vi "letak-cube.vi"   [LabVIEW 2016, in "Moving Motor.lvrbt"]
uses:
  Moving Motor.lvrbt
  <vilib>/NXT/Hardware/Plugins/Tetrix 180 deg Servo/Tetrix180ServoAddress.ctl
  <vilib>/NXT/Hardware/Plugins/Tetrix DC Motor/TetrixDCMotorAddress.ctl
  <vilib>/NXT/NXTIO Xnodes/NXTIONodeSubVIs/TETRIX IO Move Servos.vi
  <vilib>/NXT/NXTIO Xnodes/NXTIONodeSubVIs/TETRIX IO Move DC Motors.vi
  <vilib>/NXT/Dual Mode Library/Waits/Wait_Num(msec).vi
  <vilib>/NXT/NXTIO Xnodes/NXTIONodeSubVIs/TETRIX IO Stop DC Motors.vi
  <vilib>/NXT/NXTIO Xnodes/NXTIONodeSubVIs/LEGOStopAllMotors.vi
  <vilib>/NXT/Subs/LVHSConnector.ctl
  <vilib>/NXT/NXTIO Xnodes/AddressXNode/NXTIOAddress.xnode
  <vilib>/NXT/NXTIO Xnodes/NXTIOXNode/NXTIO.xnode
  <vilib>/NXT/LegoClasses/BrickReference/BrickReference.lvclass
types:
  T1 = typedef "Tetrix180ServoAddress.ctl" = i32
  T2 = cluster{"Tetrix180Servo":T1, "Tetrix180Servo":T1}
  T3 = typedef "LVHSConnector.ctl" = refnum<class "BrickReference.lvclass">
  T4 = typedef "TetrixDCMotorAddress.ctl" = i32
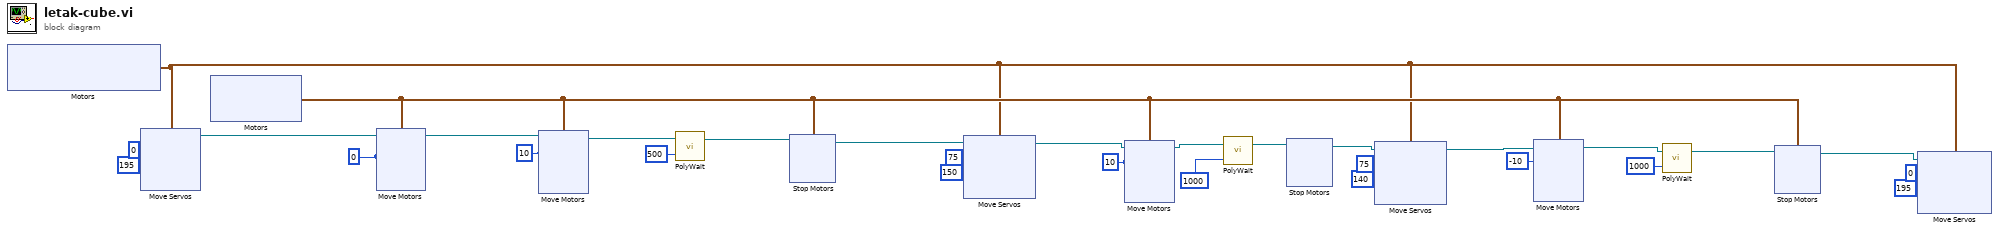
[diagram p0: block diagram]
diagram:
  w13 = i8 -10 ("Power/Speed 1")
  w16 = i8 10 ("Power/Speed 1")
  w26 = i8 10 ("Power/Speed 1")
  w28 = i8 0 ("Power/Speed 1")
  n1 = xnode "Motors"() -> ("Motor"=w4:T2)
  n2 = xnode "Move Servos"("Position 2"=u8 195, "Position 1"=u8 0, "Motors"=w4) -> ("NXT/EV3"=w27:T3)  [unwired: 1 in]
  n3 = xnode "Motors"() -> ("Motor"=w6:cluster{"TetrixDCMotor":T4, "TetrixDCMotor":T4})
  n4 = xnode "Move Motors"("Power/Speed 2"=w28, "Power/Speed 1"=w28, "Motors"=w6, "NXT/EV3"=w27) -> ("NXT/EV3"=w23:T3)
  n5 = xnode "Move Motors"("Power/Speed 2"=w26, "Power/Speed 1"=w26, "Motors"=w6, "NXT/EV3"=w23) -> ("NXT/EV3"=w24:T3)
  n6 = call-poly <vilib>:"PolyWait.vi"("Time (100 msec)"=u32 500, "NXT/EV3"=w24) -> ("NXT/EV3"=w22:T3)  [unwired: 2 in]
  n7 = xnode "Stop Motors"("Motors"=w6, "NXT/EV3"=w22) -> ("NXT/EV3"=w21:T3)
  n8 = xnode "Move Servos"("Position 2"=u8 150, "Position 1"=u8 75, "Motors"=w4, "NXT/EV3"=w21) -> ("NXT/EV3"=w14:T3)
  n9 = xnode "Move Motors"("Power/Speed 2"=w16, "Power/Speed 1"=w16, "Motors"=w6, "NXT/EV3"=w14) -> ("NXT/EV3"=w11:T3)
  n10 = call-poly <vilib>:"PolyWait.vi"("Time (100 msec)"=u32 1000, "NXT/EV3"=w11) -> ("NXT/EV3"=w10:T3)  [unwired: 2 in]
  n11 = xnode "Stop Motors"("NXT/EV3"=w10) -> ("NXT/EV3"=w9:T3)  [unwired: 1 in]
  n12 = xnode "Move Servos"("Position 2"=u8 140, "Position 1"=u8 75, "Motors"=w4, "NXT/EV3"=w9) -> ("NXT/EV3"=w12:T3)
  n13 = xnode "Move Motors"("Power/Speed 2"=w13, "Power/Speed 1"=w13, "Motors"=w6, "NXT/EV3"=w12) -> ("NXT/EV3"=w8:T3)
  n14 = call-poly <vilib>:"PolyWait.vi"("Time (100 msec)"=u32 1000, "NXT/EV3"=w8) -> ("NXT/EV3"=w5:T3)  [unwired: 2 in]
  n15 = xnode "Stop Motors"("Motors"=w6, "NXT/EV3"=w5) -> ("NXT/EV3"=w3:T3)
  n16 = xnode "Move Servos"("Position 2"=u8 195, "Position 1"=u8 0, "Motors"=w4, "NXT/EV3"=w3) -> ()  [unwired: 1 out]
